vi "Open.vi"(8 "error in (no error)":errorcluster, 11 "MelsecTCP in":refnum<class "InovanceSerial.lvclass">) -> (0 "error out":errorcluster, 3 "MelsecTCP out":refnum<class "InovanceSerial.lvclass">)   [LabVIEW 2020, in "HslCommunication.lvlib" / "InovanceSerial.lvclass"]
uses:
  InovanceSerial.lvclass
  D:/Git/Labview-Libraries/Libraries/HslCommunication/Abstract PLC Controler/Abstract PLC Controler.lvclass
  EventLogger.lvlibp/1abvi3w/vi.lib/gpm_packages/@cs/event-logger/Source/Composed Log/Types/Log Level.ctl
  InovanceSerial.lvclass/InovanceSerial.ctl
  Abstract PLC Controler/Abstract PLC Controler.lvclass/Abstract PLC Controler.ctl
  D:/Git/Labview-Libraries/Libraries/HslCommunication/_Dependenciecs/HslCommunication.dll
  _Dependenciecs/HslCommunication.dll
  Abstract PLC Controler/Abstract PLC Controler.lvclass
  EventLogger.lvlibp/Logger.lvclass
  EventLogger.lvlibp/1abvi3w/vi.lib/gpm_packages/@cs/event-logger/Source/Composed Log/Composed Log.lvlib
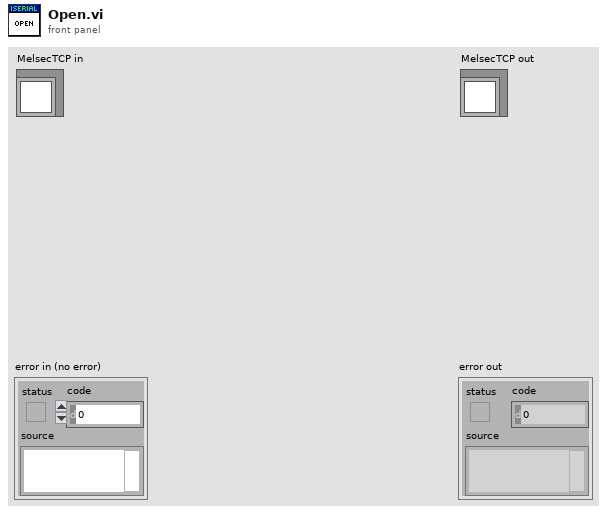
[diagram p1: front panel]
types:
  T1 = typedef "EventLogger.lvlibp/Composed Log.lvlib/Log Level.ctl" = enum16{"Debug", "Info", "Warning", "Error", "Critical"}
  T2 = cluster{"portName":string, "baudRate":i32, "dataBits":i32, "stopBits":i32, "parity":i32}
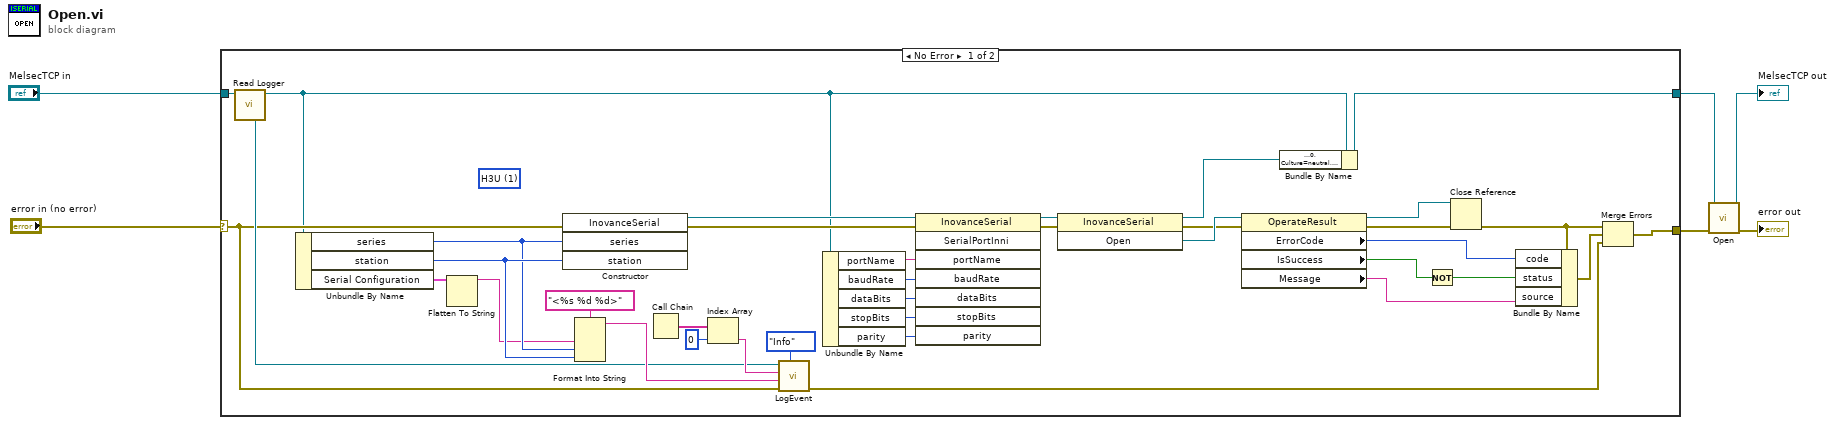
[diagram p0: block diagram]
diagram:
  n1 = case shown="No Error" "error in (no error)" {
    selector: "error in (no error)" -> [w23 w45]
    tunnel: "MelsecTCP in" -> [w43 w44]
    tunnel: [w42 w44] -> w2
    tunnel: [w36 w45] -> w4
    frame No Error {
      (unwired) 1 items=["AM", "H3U", "H5U"] ("series")
      n2 = call "Read Logger.vi"("Abstract PLC Controler in"=w43) -> ("EventLogger.lvlibp:Logger.lvclass"=w24:refnum<class "Logger.lvclass">, "Abstract PLC Controler out"=w15:refnum<class "InovanceSerial.lvclass">)  [unwired: 9 in]
      n3 = Unbundle By Name(w15) -> ("series"=w9:i32, "station"=w16:u8, "Serial Configuration"=w8:T2)
      n4 = Flatten To String(anything=w8) -> (data string=w7:string)  [unwired: 3 in, 2 out]
      n5 = constructor class="InovanceSerial"(error in=w23, "series"=w9, "station"=w16) -> (reference out=w33:refnum<k24>, error out=w32:errorcluster)  [unwired: 2 in, 3 out]
      n6 = Format Into String(format string="<%s %d %d>", w7, w9, w16) -> (resulting string=w26:string)  [unwired: 2 in, 1 out]
      n7 = Call Chain() -> (call chain=w29:string[])
      n8 = Index Array(array=w29, index=0) -> (element=w25:string)
      n9 = call "LogEvent.vi"("Event Level"=Log_Level."Info", "error in (no error)"=w23, "Data To Log"=w26, "SourceID"=w25, "Logger in"=w24) -> ("error out"=w22:errorcluster)  [unwired: 5 in, 1 out]
      n10 = Unbundle By Name(w15) -> ("portName"=w10:string, "baudRate"=w14:i32, "dataBits"=w13:i32, "stopBits"=w12:i32, "parity"=w11:i32)
      n11 = invoke class="InovanceSerial" method="SerialPortInni"(reference=w33, error in=w32, "portName"=w10, "baudRate"=w14, "dataBits"=w13, "stopBits"=w12, "parity"=w11) -> (reference out=w30:refnum<k24>, error out=w19:errorcluster)  [unwired: 1 in, 6 out]
      n12 = invoke class="InovanceSerial" method="Open"(reference=w30, error in=w19) -> (reference out=w20:refnum<k24>, error out=w17:errorcluster, "Open"=w18:refnum<k24>)  [unwired: 1 in]
      n13 = property class="OperateResult"(reference=w18, error in=w17) -> (reference out=w35:refnum<k24>, error out=w34:errorcluster, "ErrorCode"=w39:i32, "IsSuccess"=w31:bool, "Message"=w37:string)
      n14 = Bundle By Name(cluster=w15, "reference"=w20) -> (w42:refnum<class "InovanceSerial.lvclass">)
      n15 = Not(x=w31) -> (.not. x?=w38:bool)
      n16 = Close Reference(reference=w35, error in (no error)=w34) -> (error out=w40:errorcluster)
      n17 = Bundle By Name(cluster=w40, "code"=w39, "status"=w38, "source"=w37) -> (w41:errorcluster)
      n18 = Merge Errors(w40, w41, w22) -> (w36:errorcluster)
    }
    frame Error {
    }
  }
  n19 = call-parent "Open.vi"("error in (no error)"=w4, "MelsecTCP in"=w2) -> ("error out"=→"error out":errorcluster, "MelsecTCP out"=→"MelsecTCP out":refnum<class "InovanceSerial.lvclass">)  [unwired: 8 in]
